vi "CreatePrivateEvents.vi"(8 "error in (no error)":errorcluster, 11 "DSP":refnum<class "DSP.lvclass">) -> (0 "error out":errorcluster, 3 "DSP out":refnum<class "DSP.lvclass">)   [LabVIEW 2016, in "DSP.lvclass"]
doc: "---------------------------------------------------------------\nJKI State Machine Objects™\nhttp://jki.net/state-machine-objects/\nCopyright (C) 2005-2015, JKI <info@jki.net>\nALL RIGHTS RESERVEDJKI State Machine Objects (SMO) 1.0.0.4\nJKI - JKI\nCopyright (c) 2015, JKI"
uses:
  DSP.lvclass
  Typedefs/PrivateEvents--DSP.setWaveform.ctl
  Typedefs/PrivateEvents--DSP.RunCalculation.ctl
  Typedefs/LP_Config.ctl
  DSP.lockin/Typedefs/Lockin_Config.ctl
  Typedefs/FFT_Config.ctl
  <vilib>/Analysis/4window.llb/windowTd.ctl
  <vilib>/measure/maspectr.llb/Power Spectrum and PSD Export Mode.ctl
  DSP.lvclass/DSP.ctl
  <vilib>/JKI/JKI SMO/SMO/SMO.lvclass
  <vilib>/measure/NI_MAPro.lvlib
  <vilib>/Analysis/NI_AALPro.lvlib
  DSP.lockin/DSP_lockin.lvclass
panel:
  # "For instructions on how to use the JKI State Machine Objects, examples and video tutorials, visit:\nhttp://jki.net/state-machine-objects/\n\nJKI State Machine Objects™\nhttp://jki.net/state-machine-objects/\nCopyright (C) 2005-2015, JKI <info@jki.net>\nALL RIGHTS RESERVED"
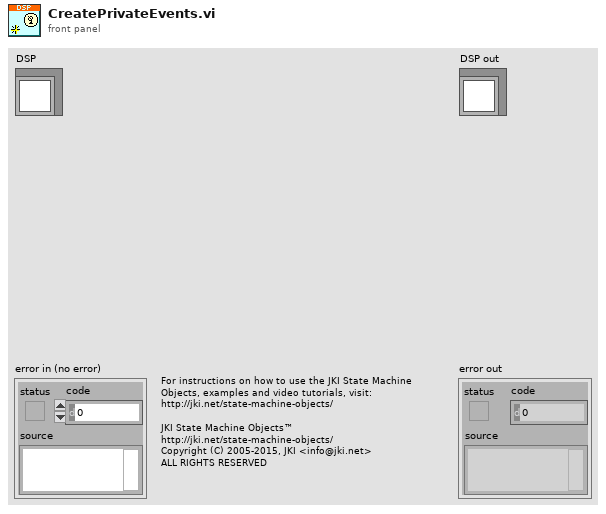
[diagram p1: front panel]
types:
  T1 = typedef "DSP.lvclass/PrivateEvents--DSP.RunCalculation.ctl" = cluster{"RunCalculation":cluster{"adjust gain":bool, "subtract offset":bool, "60 Hz prefilter":bool, "LP prefilter":bool, "lockin":bool, "FFT":bool, "gain":dbl[], "offset":dbl[], "LP config":T2, "Lockin config":T3, "FFT config":T4}}
  T2 = typedef "DSP.lvclass/LP_Config.ctl" = cluster{"high cutoff freq [Hz]":dbl}
  T3 = typedef "DSP_lockin.lvclass/Lockin_Config.ctl" = cluster{" f (Hz)":dbl, "phi (deg)":dbl, "TC (s)":dbl, "order":i32}[]
  T4 = typedef "DSP.lvclass/FFT_Config.ctl" = cluster{"averaging parameters":cluster{"averaging mode":enum16{"No averaging", "Vector averaging", "RMS averaging", "Peak hold"}, "weighting mode":enum16{"Linear", "Exponential"}, "number of averages":u32}, "window":T5, "export mode":T6, "window parameter":dbl, "restart averaging (F)":bool}
  T5 = typedef "NI_AALPro.lvlib/windowTd.ctl" = u32
  T6 = typedef "NI_MAPro.lvlib/Power Spectrum and PSD Export Mode.ctl" = u16
  T7 = typedef "PrivateEvents--DSP.setWaveform.ctl" = waveform(dbl)[]
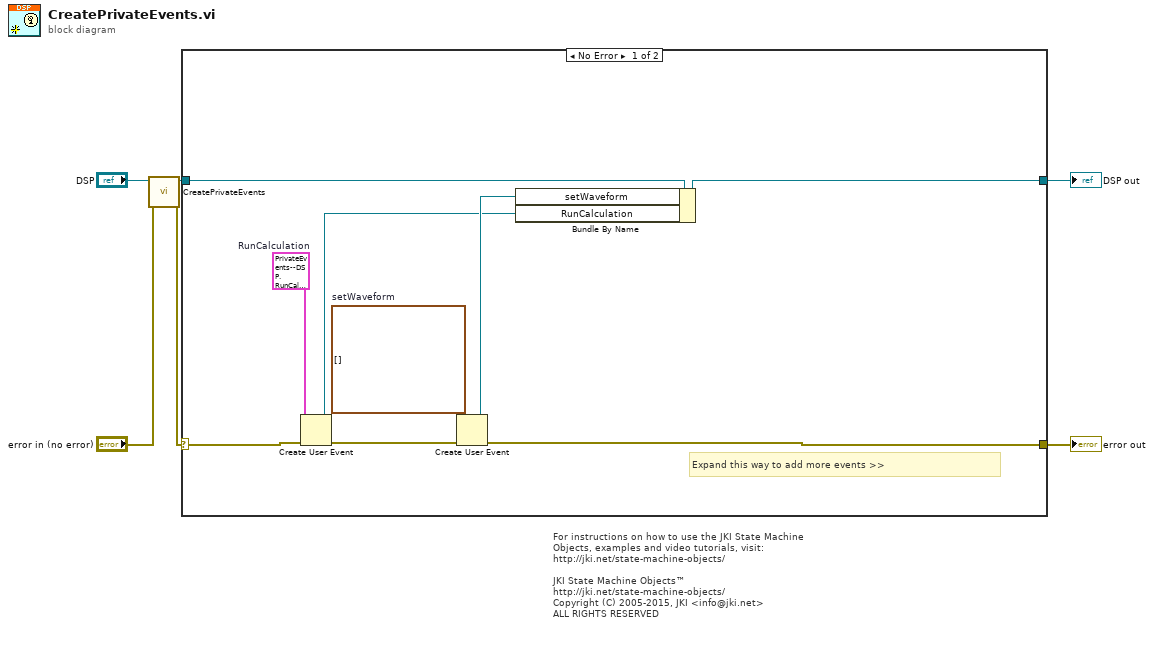
[diagram p0: block diagram]
diagram:
  # "For instructions on how to use the JKI State Machine Objects, examples and video tutorials, visit:\nhttp://jki.net/state-machine-objects/\n\nJKI State Machine Objects™\nhttp://jki.net/state-machine-objects/\nCopyright (C) 2005-2015, JKI <info@jki.net>\nALL RIGHTS RESERVED"
  n1 = call-parent "CreatePrivateEvents.vi"("error in (no error)"="error in (no error)", "SMO"="DSP") -> ("error out"=w1:errorcluster, "SMO out"=w3:refnum<class "DSP.lvclass">)  [unwired: 8 in]
  n2 = case shown="No Error" w1 {
    selector: w1 -> [w14 w17]
    tunnel: [w12 w17] -> w5
    tunnel: [w13 w16] -> w6
    tunnel: w3 -> [w15 w16]
    frame No Error {
      w8 = T1 {"RunCalculation"={"adjust gain"=FALSE, "subtract offset"=FALSE, "60 Hz prefilter"=FALSE, "LP prefilter"=FALSE, "lockin"=FALSE, "FFT"=FALSE, "gain"=[], "offset"=[], "LP config"={"high cutoff freq [Hz]"=0.0}, "Lockin config"=[], "FFT config"={"averaging parameters"={"averaging mode"=enum."No averaging", "weighting mode"=enum."Linear", "number of averages"=0}, "window"=0, "export mode"=0, "window parameter"=0.0, "restart averaging (F)"=FALSE}}}  # RunCalculation
      w11 = T7 []  # setWaveform
      # "Expand this way to add more events >>"
      n3 = Create User Event(user event datatype=w8, error in=w14) -> (user event=w7:refnum<user-event>, error out=w9:errorcluster)
      n4 = Create User Event(user event datatype=w11, error in=w9) -> (user event=w10:refnum<user-event>, error out=w12:errorcluster)
      n5 = Bundle By Name(cluster=w15, "setWaveform"=w10, "RunCalculation"=w7) -> (w13:refnum<class "DSP.lvclass">)
    }
    frame Error {
    }
  }
  "error out" <- w5
  "DSP out" <- w6
